vi "Set Zero Offset Mode.vi"(8 "error in (no error)":errorcluster, 9 "Reference Value (0.0)":dbl format="%.4f", 10 "Zero Offset Mode (F: Off)":bool, 11 "VISA resource name":refnum<visa-resource-name>) -> (0 "error out":errorcluster, 3 "VISA resource name out":refnum<visa-resource-name>)   [LabVIEW 2011, in "Fluke 5XXX Series Multicalibrators.lvlib"]
doc: "This VI zeros the pressure module or sets the zero offset for capacitance measurement using the oscilloscope option. For pressure measurments, if the pressure module is an absolute module, the reference parameter must be supplied.\n\nNote:\n\nThis VI is available only for instrument models 5500A and 5520A with oscilloscope option SC600 (SC1100) or option 700P (pressure modules)."
uses:
  Fluke 5XXX Series Multicalibrators.lvlib
panel:
  # "On"
  # "Off"
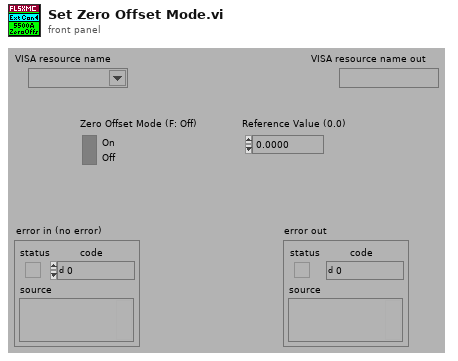
[diagram p1: front panel]
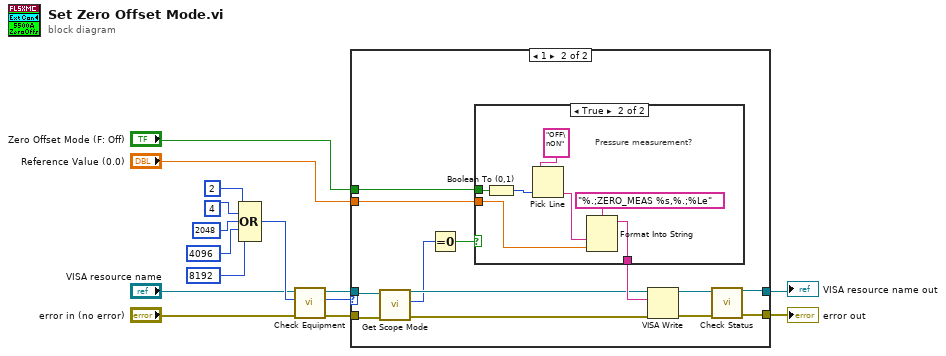
[diagram p0: block diagram]
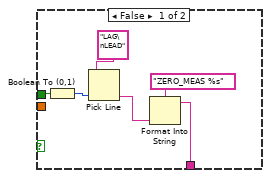
[diagram p3: hidden frame]
diagram:
  n1 = Compound Arithmetic op=OR(2 ("Numeric"), 4 ("Numeric"), 2048 ("Numeric"), 4096 ("Numeric"), 8192 ("Numeric")) -> (w8:i32)
  n2 = call "Check Equipment.vi"("error in (no error)"="error in (no error)", "Bit Mask"=w8, "VISA resource name"="VISA resource name") -> ("error out"=w15:errorcluster, "Present?"=w14:u32, "VISA resource name out"=w13:refnum<visa-resource-name>)  [unwired: 6 in]
  n3 = case shown="1" w14 {
    tunnel: [w16 w27] -> w3
    tunnel: w15 -> [w17 w22]
    tunnel: w13 -> [w16 w23]
    tunnel: [w17 w30] -> w4
    tunnel: "Zero Offset Mode (F: Off)" -> [_ w19]
    tunnel: "Reference Value (0.0)" -> [_ w18]
    frame 0, Default {
    }
    frame 1 {
      n4 = call "Get Scope Mode.vi"("error in (no error)"=w22, "VISA resource name"=w23) -> ("error out"=w25:errorcluster, "Scope Mode"=w21:i32, "VISA resource name out"=w24:refnum<visa-resource-name>)  [unwired: 7 in]
      n5 = Equal To 0?(x=w21) -> (x = 0?=w20:bool)
      n6 = case shown="True" w20 {
        tunnel: [w35 w37] -> w26
        tunnel: w19 -> [w32 w39]
        tunnel: w18 -> [_ w41]
        frame False {
          n7 = Boolean To (0,1)(Boolean=w32) -> (0, 1=w31:i16)
          n8 = Pick Line(multi-line string="LAG\nLEAD", line index=w31) -> (output string=w33:string)  [unwired: 1 in]
          n9 = Format Into String(format string="ZERO_MEAS %s", w33) -> (resulting string=w35:string)  [unwired: 2 in, 1 out]
        }
        frame True {
          # "Pressure measurement?"
          n10 = Boolean To (0,1)(Boolean=w39) -> (0, 1=w38:i16)
          n11 = Pick Line(multi-line string="OFF\nON", line index=w38) -> (output string=w40:string)  [unwired: 1 in]
          n12 = Format Into String(format string="%.;ZERO_MEAS %s,%.;%Le", w40, w41) -> (resulting string=w37:string)  [unwired: 2 in, 1 out]
        }
      }
      n13 = VISA Write(VISA resource name=w24, write buffer=w26, error in (no error)=w25) -> (VISA resource name out=w28:refnum<visa-resource-name>, error out=w29:errorcluster)  [unwired: 1 out]
      n14 = call "Check Status.vi"("VISA resource name"=w28, "error in (no error)"=w29) -> ("VISA resource name out"=w27:refnum<visa-resource-name>, "error out"=w30:errorcluster)  [unwired: 12 in]
    }
  }
  "VISA resource name out" <- w3
  "error out" <- w4
